vi "libssh2_userauth_publickey_frommemory.vi"(5 "private key data":string, 7 "public key data":string, 8 "error in (no error)":errorcluster, 9 "passphrase":string, 10 "username":string, 11 "session":T1) -> (0 "error out":errorcluster)   [LabVIEW 2013, in "libssh2.lvlib"]
doc: "Authenticate a session using a private and public key from memory."
uses:
  libssh2.lvlib
  Session Refnum.ctl
  Not A Session.vi
  <vilib>/Utility/error.llb/Error Cluster From Error Code.vi
  Global Settings.vi
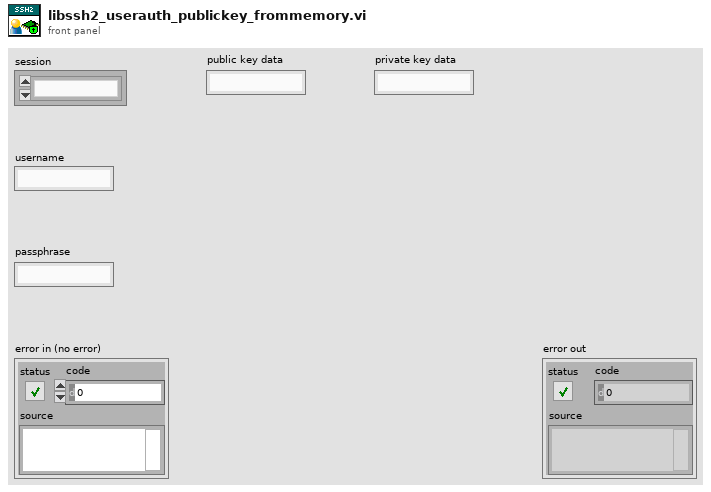
[diagram p1: front panel]
types:
  T1 = typedef "libssh2.lvlib/Session Refnum.ctl" = refnum<k1>
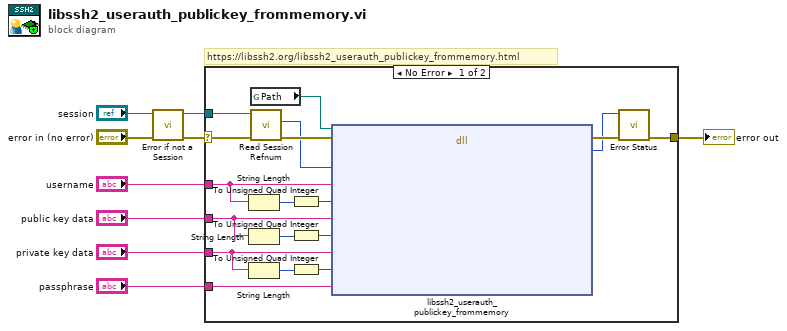
[diagram p0: block diagram]
diagram:
  # "https://libssh2.org/libssh2_userauth_publickey_frommemory.html"
  n1 = call "Error if not a Session.vi"("error in (no error)"="error in (no error)", "session"="session") -> ("error out"=w6:errorcluster, "session out"=w4:T1)  [unwired: 8 in]
  n2 = case shown="No Error" w6 {
    selector: w6 -> [w26 w28]
    tunnel: "username" -> [w27 _]
    tunnel: [w25 w28] -> w8
    tunnel: w4 -> [w24 _]
    tunnel: "public key data" -> [w10 _]
    tunnel: "private key data" -> [w11 _]
    tunnel: "passphrase" -> [w16 _]
    frame No Error {
      n3 = String Length(string=w27) -> (length=w21:i32)
      n4 = String Length(string=w10) -> (length=w15:i32)
      n5 = String Length(string=w11) -> (length=w14:i32)
      n6 = global read "Global Settings.vi" "Path"() -> (w18:path)
      n7 = call "Read Session Refnum.vi"("error in (no error)"=w26, "session"=w24) -> ("error out"=w20:errorcluster, "LIBSSH2_SESSION*"=w19:u64)  [unwired: 5 in, 3 out]
      n8 = To Unsigned Quad Integer(1:w21) -> (0:w23:u64)
      n9 = To Unsigned Quad Integer(1:w15) -> (0:w12:u64)
      n10 = To Unsigned Quad Integer(1:w14) -> (0:w13:u64)
      n11 = dll-call lib="?" fn="libssh2_userauth_publickey_frommemory"(path in=w18, error in=w20, "session"=w19, "username"=w27, "username_len"=w23, "publickeyfiledata"=w10, "publickeyfiledata_len"=w12, "privatekeyfiledata"=w11, "privatekeyfiledata_len"=w13, "passphrase"=w16) -> (error out=w22:errorcluster, "return value"=w17:i32)  [unwired: 9 in, 1 out]
      n12 = call "Error Status.vi"("error in (no error)"=w22, "return value"=w17) -> ("error out"=w25:errorcluster)  [unwired: 8 in, 1 out]
    }
    frame Error {
    }
  }
  "error out" <- w8
